vi "Clear Attacked.vi"(11 "Array in":T1[][](array[typedef])) -> (3 "Array out":T1[][](array[typedef]))   [LabVIEW 2014, in "SquareBattle Arena.lvlib" / "SquareBattle Arena.lvclass"]
uses:
  SquareBattle Arena.lvclass
  Runner Cluster.ctl
  Square/Square.lvclass
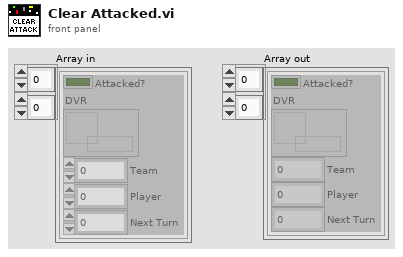
[diagram p1: front panel]
types:
  T1 = typedef "SquareBattle Arena.lvlib/SquareBattle Arena.lvclass/Runner Cluster.ctl" = cluster{"Attacked?":bool, "DVR":refnum<data-value>, "Team":i32, "Player":i32, "Next Turn":i32}
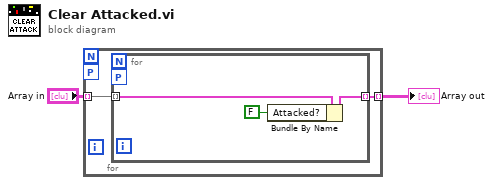
[diagram p0: block diagram]
diagram:
  n1 = for {
    tunnel: "Array in" -> [w4] mode=indexing
    tunnel: [w3] -> w2 mode=indexing
    workers-P: _ -> [_]
    n2 = for {
      tunnel: w4 -> [w6] mode=indexing
      tunnel: [w7] -> w3 mode=indexing
      workers-P: _ -> [_]
      n3 = Bundle By Name(cluster=w6, "Attacked?"=FALSE) -> (w7:T1)
    }
  }
  "Array out" <- w2
